vi "BothArmsPosition.vi"(0 "error in":errorcluster, 2 "Parameters":T1 {"left_w2" scale=-180.0..180.0; "left_w1" scale=-180.0..180.0; "left_w0" scale=-180.0..180.0; "left_e1" scale=-180.0..180.0; "left_e0" scale=-180.0..180.0; "left_s1" scale=-180.0..180.0; "left_s0" scale=-180.0..180.0; "right_s1" scale=-180.0..180.0; "right_s0" scale=-180.0..180.0; "right_w2" scale=-180.0..180.0; "right_e1" scale=-180.0..180.0; "right_e0" scale=-180.0..180.0; "right_w0" scale=-180.0..180.0; "right_w1" scale=-180.0..180.0}, 3 "node":string) -> (1 "error out":errorcluster)   [LabVIEW 2015]
doc: "This VI moves both the Baxter arms to a given position."
uses:
  ROS/Code/JointPositions.ctl
  ROS/Code/Slider.ctl
  ROS/Code/SubVIs/BaxterSide.ctl
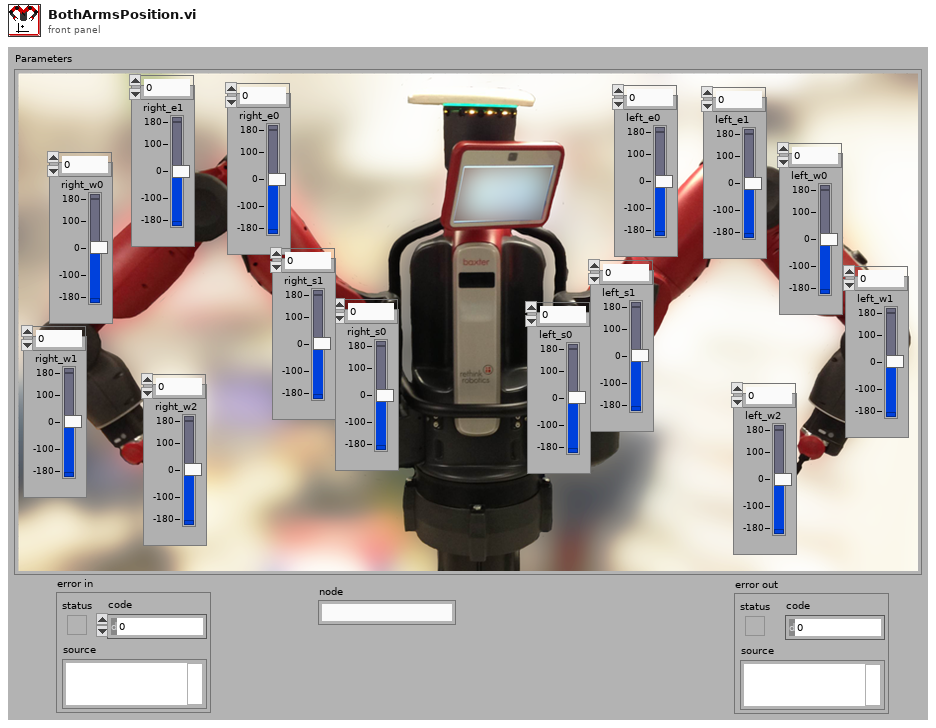
[diagram p1: front panel]
types:
  T1 = typedef "JointPositions.ctl" = cluster{"left_e0":T2, "left_e1":T2, "left_s0":T2, "left_s1":T2, "left_w0":T2, "left_w1":T2, "left_w2":T2, "right_e0":T2, "right_e1":T2, "right_s0":T2, "right_s1":T2, "right_w0":T2, "right_w1":T2, "right_w2":T2}
  T2 = typedef "Slider.ctl" = dbl
  T3 = typedef "BaxterSide.ctl" = enum16{"left", "right"}
  T4 = cluster{"[0]":T2, "[1]":T2, "[2]":T2, "[3]":T2, "[4]":T2, "[5]":T2, "[6]":T2}
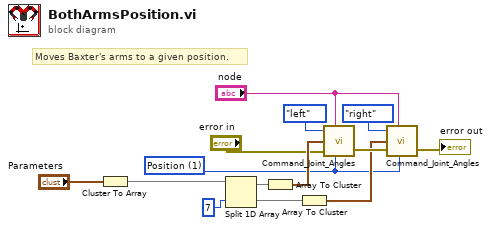
[diagram p0: block diagram]
diagram:
  w2 = u8 1 items=["Position"=1, "Velocity"=2, "Effort"=3] ("Mode")
  # "Moves Baxter's arms to a given position."
  n1 = Cluster To Array(cluster="Parameters") -> (array=w3:T2[])
  n2 = Split 1D Array(array=w3, index=7) -> (first subarray=w7:T2[], second subarray=w6:T2[])
  n3 = Array To Cluster(array=w7) -> (cluster=w5:T4)
  n4 = Array To Cluster(array=w6) -> (cluster=w4:T4)
  n5 = call "Command_Joint_Angles.vi"("Side"=BaxterSide."left", "node"="node", "Arm Angles (degrees)"=w5, "error in"="error in", "Mode"=w2) -> ("error out"=w12:errorcluster)  [unwired: 1 in]
  n6 = call "Command_Joint_Angles.vi"("Side"=BaxterSide."right", "node"="node", "Arm Angles (degrees)"=w4, "error in"=w12, "Mode"=w2) -> ("error out"=→"error out":errorcluster)  [unwired: 1 in]
